vi "Destructor.vi"(8 "error in":errorcluster, 11 "StepRun":refnum<class "StepRun.lvclass">) -> (0 "error out":errorcluster)   [LabVIEW 2021, in "ProligentXMLGenerator.lvlib" / "StepRun.lvclass"]
uses:
  StepRun.lvclass
  StepRun.lvclass/StepRun.ctl
  Measure/RealMeasure/RealMeasure.lvclass
  Measure/StringMeasure/StringMeasure.lvclass
  Measure/BooleanMeasure/BooleanMeasure.lvclass
  Measure/IntegerMeasure/IntegerMeasure.lvclass
  Measure/DateTimeMeasure/DateTimeMeasure.lvclass
  Model/Characteristic/Characteristic.lvclass
  Measure/Measure/Measure.lvclass
  Failure/FailureReference/FailureReference.lvclass
  Model/Document/Document.lvclass
  Model/CustomData/CustomData.lvclass
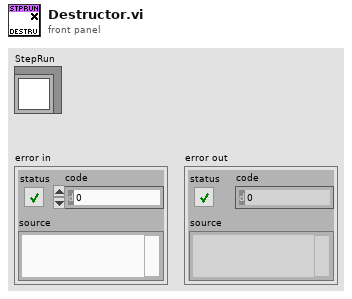
[diagram p1: front panel]
types:
  T1 = typedef "ProligentXMLGenerator.lvlib/StepRun.lvclass/Data.ctl" = cluster{"Name":string, "Measures":refnum<class "Measure.lvclass">[], "FailureReferences":refnum<class "FailureReference.lvclass">[], "Characteristics":refnum<class "Characteristic.lvclass">[], "Documents":refnum<class "Document.lvclass">[], "CustomData":refnum<class "CustomData.lvclass">, "StepExecutionStatus":refnum<class "ExecutionStatus.lvclass">, "StepRunId":refnum<class "Guid.lvclass">, "StepName":refnum<class "NonEmptyString_255.lvclass">, "StartDate":refnum<class "DateTime.lvclass">, "EndDate":refnum<class "DateTime.lvclass">, "TimeZoneInfoId":string}
  T2 = typedef "ProligentXMLGenerator.lvlib/MeasureKind.lvclass/Value.ctl" = enum16{"REAL", "BOOL", "INTEGER", "STRING", "DATETIME"}
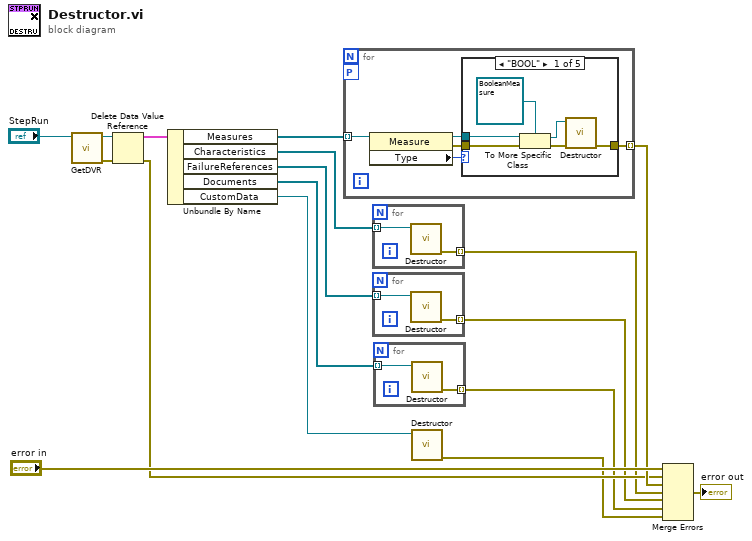
[diagram p0: block diagram]
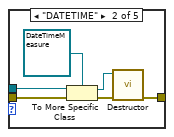
[diagram p2: hidden frame]
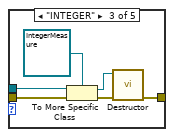
[diagram p3: hidden frame]
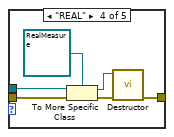
[diagram p4: hidden frame]
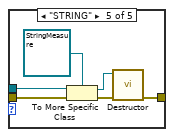
[diagram p5: hidden frame]
diagram:
  n1 = call "GetDVR.vi"("StepRun"="StepRun") -> ("error out"=w14:errorcluster, "DVRReference"=w15:refnum<data-value>)  [unwired: 9 in]
  n2 = Delete Data Value Reference(data value reference=w15, error in=w14) -> (data value=w13:T1, error out=w9:errorcluster)
  n3 = Unbundle By Name(w13) -> ("Measures"=w10:refnum<class "Measure.lvclass">[], "Characteristics"=w8:refnum<class "Characteristic.lvclass">[], "FailureReferences"=w6:refnum<class "FailureReference.lvclass">[], "Documents"=w3:refnum<class "Document.lvclass">[], "CustomData"=w2:refnum<class "CustomData.lvclass">)
  n4 = for {
    tunnel: w10 -> [w22] mode=indexing
    tunnel: [w18] -> w11 mode=indexing
    workers-P: _ -> [_]
    n5 = property on="Property Node" class="Measure"(reference=w22) -> (reference out=w20:refnum<class "Measure.lvclass">, error out=w21:errorcluster, "Type"=w19:T2)  [unwired: 1 in]
    n6 = case shown="\"BOOL\"" w19 {
      tunnel: w21 -> [w28 w34 w40 w46 w52]
      tunnel: w20 -> [w24 w30 w36 w42 w48]
      tunnel: [w26 w32 w38 w44 w50] -> w18
      frame "BOOL" {
        n7 = To More Specific Class(target class=refnum<class "BooleanMeasure.lvclass"> refnum ("ProligentResultProcessor:BooleanMeasure"), reference=w24, error in=w28) -> (specific class reference=w23:refnum<class "BooleanMeasure.lvclass">, error out=w27:errorcluster)
        n8 = call "Destructor.vi"("error in"=w27, "BooleanMeasure"=w23) -> ("error out"=w26:errorcluster)  [unwired: 9 in]
      }
      frame "DATETIME" {
        n9 = To More Specific Class(target class=refnum<class "DateTimeMeasure.lvclass"> refnum ("ProligentResultProcessor:DateTimeMeasure"), reference=w30, error in=w34) -> (specific class reference=w29:refnum<class "DateTimeMeasure.lvclass">, error out=w33:errorcluster)
        n10 = call "Destructor.vi"("error in"=w33, "DateTimeMeasure"=w29) -> ("error out"=w32:errorcluster)  [unwired: 9 in]
      }
      frame "INTEGER" {
        n11 = To More Specific Class(target class=refnum<class "IntegerMeasure.lvclass"> refnum ("ProligentResultProcessor:RealMeasure"), reference=w36, error in=w40) -> (specific class reference=w35:refnum<class "IntegerMeasure.lvclass">, error out=w39:errorcluster)
        n12 = call "Destructor.vi"("error in"=w39, "IntergerMeasure"=w35) -> ("error out"=w38:errorcluster)  [unwired: 9 in]
      }
      frame "REAL" {
        n13 = To More Specific Class(target class=refnum<class "RealMeasure.lvclass"> refnum ("ProligentResultProcessor:RealMeasure"), reference=w42, error in=w46) -> (specific class reference=w41:refnum<class "RealMeasure.lvclass">, error out=w45:errorcluster)
        n14 = call "Destructor.vi"("error in"=w45, "RealMeasure"=w41) -> ("error out"=w44:errorcluster)  [unwired: 9 in]
      }
      frame "STRING" {
        n15 = To More Specific Class(target class=refnum<class "StringMeasure.lvclass"> refnum ("ProligentResultProcessor:StringMeasure"), reference=w48, error in=w52) -> (specific class reference=w47:refnum<class "StringMeasure.lvclass">, error out=w51:errorcluster)
        n16 = call "Destructor.vi"("error in"=w51, "StringMeasure"=w47) -> ("error out"=w50:errorcluster)  [unwired: 9 in]
      }
    }
  }
  n17 = for {
    tunnel: w8 -> [w54] mode=indexing
    tunnel: [w53] -> w7 mode=indexing
    n18 = call "Destructor.vi"("Document in"=w54) -> ("error out"=w53:errorcluster)  [unwired: 10 in]
  }
  n19 = for {
    tunnel: w6 -> [w56] mode=indexing
    tunnel: [w55] -> w5 mode=indexing
    n20 = call "Destructor.vi"("FailureReference in"=w56) -> ("error out"=w55:errorcluster)  [unwired: 10 in]
  }
  n21 = for {
    tunnel: w3 -> [w58] mode=indexing
    tunnel: [w57] -> w4 mode=indexing
    n22 = call "Destructor.vi"("Document in"=w58) -> ("error out"=w57:errorcluster)  [unwired: 10 in]
  }
  n23 = call "Destructor.vi"("CustomDataType"=w2) -> ("error out"=w1:errorcluster)  [unwired: 10 in]
  n24 = Merge Errors("error in", w9, w11, w7, w5, w4, w1) -> (→"error out":errorcluster)
